vi "Menu Compiler.vi"(4 "error in":errorcluster, 6 "file (use dialog)":path=path "C:/Users/Michael/Dropbox/stooge identifier.json", 7 "NotifyIcon":refnum<k24>) -> (0 "error out":errorcluster, 2 "Menu Items":refnum<k24>[](array[refnum]), 3 "NotifyIcon Out":refnum<k24>)   [LabVIEW 2020, in "NotifyIcon.lvlib"]
uses:
  NotifyIcon.lvlib
  System.Windows.Forms
  _typedefs/menu item raw definition.ctl
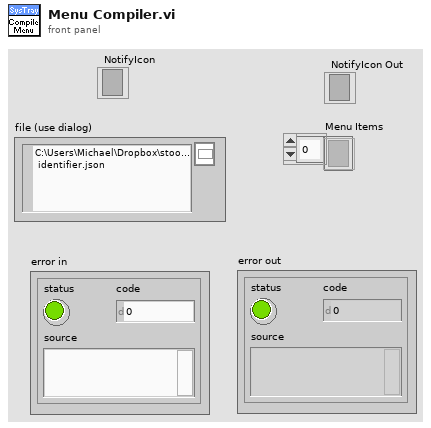
[diagram p1: front panel]
types:
  T1 = typedef "NotifyIcon.lvlib/menu item raw definition.ctl" = cluster{"Menu Order":i32, "Item Name":string, "Item Tag":string, "Parent Tag":string, "Enabled":bool}
  T2 = cluster{"Menu Level":i16, "Menu Order":i32, "Item Name":string, "Item Tag":string, "Parent Tag":string, "Enabled":bool}
  T3 = cluster{"Menu Level":i16, "Menu Order":i32, "Item Name":string, "Item Tag":string, "Parent Tag":string, "Enabled":bool}[]
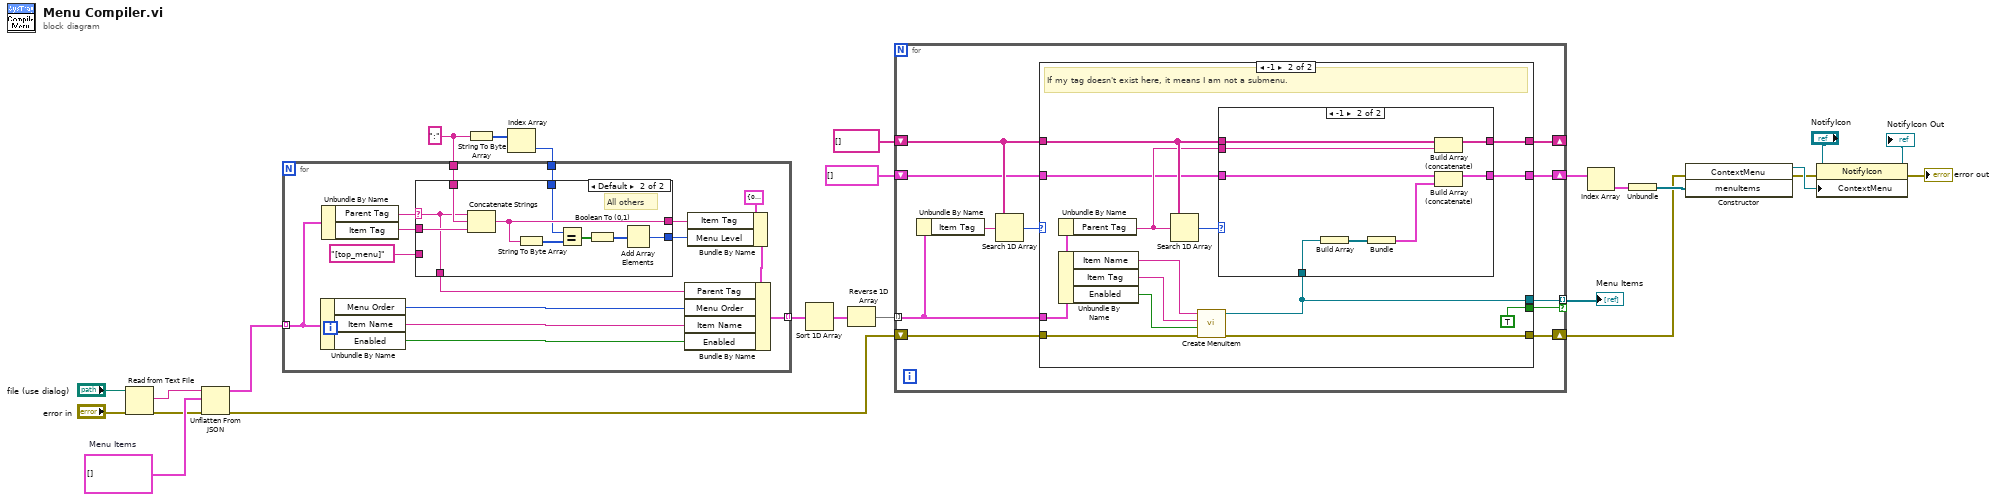
[diagram p0: block diagram]
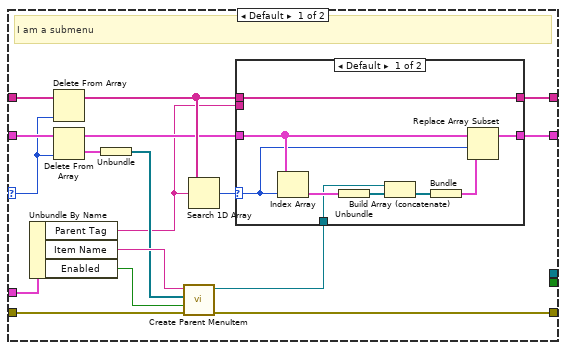
[diagram p2: hidden frame]
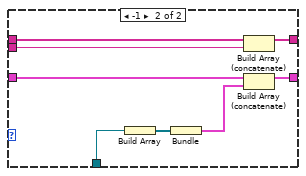
[diagram p3: hidden frame]
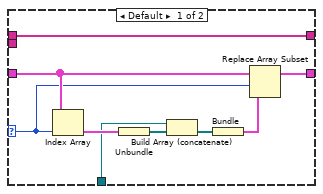
[diagram p4: hidden frame]
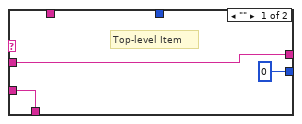
[diagram p5: hidden frame]
diagram:
  w17 = ":"
  w23 = T1[] []  # Menu Items
  n1 = Read from Text File(file (use dialog)="file (use dialog)", error in="error in") -> (text=w24:string, error out=w22:errorcluster)  [unwired: 2 in, 2 out]
  n2 = Unflatten From JSON(JSON string=w24, type and defaults=w23, error in (no error)=w22) -> (value=w20:T1[], error out=w11:errorcluster)  [unwired: 4 in]
  n3 = String To Byte Array(string=w17) -> (unsigned byte array=w18:u8[])
  n4 = Index Array(array=w18) -> (element=w16:u8)  [unwired: 1 in]
  n5 = for {
    tunnel: w20 -> [w36] mode=indexing
    tunnel: [w31] -> w19 mode=indexing
    tunnel: w17 -> [w38]
    tunnel: w16 -> [w29]
    n6 = Unbundle By Name(w36) -> ("Menu Order"=w35:i32, "Item Name"=w34:string, "Enabled"=w33:bool)
    n7 = Unbundle By Name(w36) -> ("Parent Tag"=w37:string, "Item Tag"=w39:string)
    n8 = case shown="Default" w37 {
      selector: w37 -> [_ w44]
      tunnel: w39 -> [w43 w52]
      tunnel: w38 -> [_ w51]
      tunnel: [w43 w47] -> w30
      tunnel: w29 -> [_ w46]
      tunnel: [i16 0 w45] -> w28
      tunnel: [w41 w44] -> w27
      tunnel: "[top_menu]" -> [w41 _]
      frame "" {
        # "Top-level Item"
      }
      frame Default {
        # "All others"
        n9 = Concatenate Strings(w44, w51, w52) -> (w47:string)
        n10 = String To Byte Array(string=w47) -> (unsigned byte array=w48:u8[])
        n11 = Equal?(x=w46, y=w48) -> (x = y?=w49:bool[])
        n12 = Boolean To (0,1)(Boolean=w49) -> (0, 1=w50:i16[])
        n13 = Add Array Elements(numeric array=w50) -> (sum=w45:i16)
      }
    }
    n14 = Bundle By Name(cluster=T2 {"Menu Level"=0, "Menu Order"=0, "Item Name"="", "Item Tag"="", "Parent Tag"="", "Enabled"=FALSE}, "Item Tag"=w30, "Menu Level"=w28) -> (w32:T2)
    n15 = Bundle By Name(cluster=w32, "Parent Tag"=w27, "Menu Order"=w35, "Item Name"=w34, "Enabled"=w33) -> (w31:T2)
  }
  n16 = Sort 1D Array(array=w19) -> (sorted array=w15:T3)
  n17 = Reverse 1D Array(array=w15) -> (reversed array=w14:T3)
  n18 = for {
    tunnel: w14 -> [w59] mode=indexing
    shift-right: [w61] -> _
    shift-left: string[] [] -> [w60]
    shift-right: [w57] -> w5
    shift-left: w11 -> [w58]
    shift-right: [w55] -> w8
    shift-left: cluster{refnum<k24>[]}[] [] -> [w56]
    tunnel: [w54] -> w1 mode=indexing if=w53
    n19 = Unbundle By Name(w59) -> ("Item Tag"=w63:string)
    n20 = Search 1D Array(1D array=w60, element=w63) -> (index of element=w62:i32)  [unwired: 1 in]
    n21 = case shown="-1" w62 {
      selector: w62 -> [w73 _]
      tunnel: [w69 w104] -> w61
      tunnel: w60 -> [w75 w105]
      tunnel: w59 -> [w79 w106]
      tunnel: w58 -> [w80 w111]
      tunnel: [w64 w100] -> w57
      tunnel: w56 -> [w74 w102]
      tunnel: [w68 w101] -> w55
      tunnel: [_ w99] -> w54
      tunnel: [_ TRUE] -> w53
      frame Default {
        # "I am a submenu"
        n22 = Unbundle By Name(w79) -> ("Parent Tag"=w66:string, "Item Name"=w77:string, "Enabled"=w78:bool)
        n23 = Delete From Array(array=w75, index=w73) -> (array with subset deleted=w70:string[])  [unwired: 1 in, 1 out]
        n24 = Delete From Array(array=w74, index=w73) -> (deleted portion=w72:cluster{refnum<k24>[]}, array with subset deleted=w67:cluster{refnum<k24>[]}[])  [unwired: 1 in]
        n25 = Unbundle(w72) -> (w76:refnum<k24>[])
        n26 = call "Create Parent MenuItem.vi"("error in (no error)"=w80, "Enabled"=w78, "Child MenuItems"=w76, "Item Text"=w77) -> ("error out"=w64:errorcluster, "MenuItem"=w65:refnum<k24>)  [unwired: 2 in]
        n27 = Search 1D Array(1D array=w70, element=w66) -> (index of element=w71:i32)  [unwired: 1 in]
        n28 = case shown="Default" w71 {
          selector: w71 -> [w81 _]
          tunnel: w70 -> [w84 w95]
          tunnel: [w84 w94] -> w69
          tunnel: [w83 w93] -> w68
          tunnel: w67 -> [w85 w92]
          tunnel: w66 -> [_ w91]
          tunnel: w65 -> [w82 w90]
          frame Default {
            n29 = Index Array(array=w85, index=w81) -> (element=w86:cluster{refnum<k24>[]})
            n30 = Unbundle(w86) -> (w87:refnum<k24>[])
            n31 = Build Array (concatenate)(w82, w87) -> (w88:refnum<k24>[])
            n32 = Bundle(w88) -> (w89:cluster{refnum<k24>[]})  [unwired: 1 in]
            n33 = Replace Array Subset(array=w85, new element=w89, index=w81) -> (w83:cluster{refnum<k24>[]}[])
          }
          frame -1 {
            n34 = Build Array(w90) -> (w97:refnum<k24>[])
            n35 = Bundle(w97) -> (w96:cluster{refnum<k24>[]})  [unwired: 1 in]
            n36 = Build Array (concatenate)(w95, w91) -> (w94:string[])
            n37 = Build Array (concatenate)(w92, w96) -> (w93:cluster{refnum<k24>[]}[])
          }
        }
      }
      frame -1 {
        # "If my tag doesn't exist here, it means I am not a submenu."
        n38 = Unbundle By Name(w106) -> ("Parent Tag"=w103:string)
        n39 = Unbundle By Name(w106) -> ("Item Name"=w110:string, "Item Tag"=w109:string, "Enabled"=w108:bool)
        n40 = Search 1D Array(1D array=w105, element=w103) -> (index of element=w107:i32)  [unwired: 1 in]
        n41 = call "Create MenuItem.vi"("error in (no error)"=w111, "Enabled"=w108, "Item Tag"=w109, "Item Text"=w110) -> ("error out"=w100:errorcluster, "MenuItem out"=w99:refnum<k24>)  [unwired: 2 in]
        n42 = case shown="-1" w107 {
          selector: w107 -> [w115 _]
          tunnel: w105 -> [w120 w128]
          tunnel: [w120 w126] -> w104
          tunnel: w103 -> [_ w127]
          tunnel: w102 -> [w117 w125]
          tunnel: [w116 w124] -> w101
          tunnel: w99 -> [w112 w121]
          frame Default {
            n43 = Index Array(array=w117, index=w115) -> (element=w119:cluster{refnum<k24>[]})
            n44 = Unbundle(w119) -> (w118:refnum<k24>[])
            n45 = Build Array (concatenate)(w112, w118) -> (w114:refnum<k24>[])
            n46 = Bundle(w114) -> (w113:cluster{refnum<k24>[]})  [unwired: 1 in]
            n47 = Replace Array Subset(array=w117, new element=w113, index=w115) -> (w116:cluster{refnum<k24>[]}[])
          }
          frame -1 {
            n48 = Build Array(w121) -> (w123:refnum<k24>[])
            n49 = Bundle(w123) -> (w122:cluster{refnum<k24>[]})  [unwired: 1 in]
            n50 = Build Array (concatenate)(w128, w127) -> (w126:string[])
            n51 = Build Array (concatenate)(w125, w122) -> (w124:cluster{refnum<k24>[]}[])
          }
        }
      }
    }
  }
  "Menu Items" <- w1
  n52 = Index Array(array=w8) -> (element=w7:cluster{refnum<k24>[]})  [unwired: 1 in]
  n53 = Unbundle(w7) -> (w6:refnum<k24>[])
  n54 = constructor class="ContextMenu"(error in=w5, "menuItems"=w6) -> (reference out=w10:refnum<k24>, error out=w9:errorcluster)  [unwired: 2 in, 2 out]
  n55 = property class="NotifyIcon"(reference="NotifyIcon", error in=w9, "ContextMenu"=w10) -> (reference out=→"NotifyIcon Out":refnum<k24>, error out=→"error out":errorcluster)
